vi "GeneratePhaseCUDAv2.vi"() -> ()   [LabVIEW 2019]
uses:
  <vilib>/imath/engines/lvmath2/RunTimeEngine/RangeToken/NIMS_Range.vi
  <instcachedir>/0/NIMS_Range_0856D726B6B24596B614846B21C682A9.lvgen/NIMS_Range_0856D726B6B24596B614846B21C682A9_001.vi
  <vilib>/imath/engines/lvmath2/RunTimeEngine/BuiltInFunctions/meshgrid2d/NIMS_meshgrid2d(V,V).vi
  <instcachedir>/0/NIMS_meshgrid2d(V,V)_3733343E1C554A708015CFB0432C6A59.lvgen/NIMS_meshgrid2d(V,V)_3733343E1C554A708015CFB0432C6A59_000.vi
  <vilib>/imath/engines/lvmath2/RunTimeEngine/ErrorHandling/NIMS_Create Error From Enums.vi
  <vilib>/imath/engines/lvmath2/RunTimeEngine/IndexRead/NIMS M($).vi
  <instcachedir>/0/NIMS M($)_82D1177398184AFB96A6AFB63C3C3F57.lvgen/NIMS M($)_82D1177398184AFB96A6AFB63C3C3F57_000.vi
  <vilib>/imathl/engines/lvmath/Functions/Error Handling/Create Error.vi
  <vilib>/imath/engines/lvmath2/RunTimeEngine/BuiltInFunctions/length/NIMS_length(GV).vi
  <instcachedir>/0/NIMS_length(GV)_08A3D13377FD4E4B96F5795FBF3698FA.lvgen/NIMS_length(GV)_08A3D13377FD4E4B96F5795FBF3698FA_000.vi
  <vilib>/imath/engines/lvmath2/RunTimeEngine/BuiltInFunctions/zeros/NIMS_V=zeros(I32,I32).vi
  <vilib>/imath/engines/lvmath2/RunTimeEngine/BuiltInFunctions/ones/NIMS_V=ones(I32,I32).vi
  <vilib>/imath/engines/lvmath2/RunTimeEngine/NodeEndStatement/NIMS_NodeEndStatement_Output.vi
  <instcachedir>/0/NIMS_NodeEndStatement_Output_53EC0D466D134D7ABD903AC30B43404B.lvgen/NIMS_NodeEndStatement_Output_53EC0D466D134D7ABD903AC30B43404B_005.vi
  <vilib>/imath/engines/lvmath2/RunTimeEngine/ErrorHandling/NIMS_Finalize Error.vi
  PCIe16LabVIEWSDK/Interface.dll
panel:
  out "Delay [ms] 2":dbl
  out "board 2":i32
  out "generatePhase Return 2":i32
  in  "I0":dbl=1.0
  in  "y0":i32
  in  "x0":i32
  in  "dy":i32=24
  in  "dx":i32=24
  in  "ny":i32=12
  in  "nx":i32=12
  in  "Generate":bool
  out "Y Array":sgl[](array[numeric])
  out "X Array":sgl[](array[numeric])
  out "board":i32
  in  "Start SLM":bool
  out "Board ID":i32
  out "# of Boards":i32
  in  "SLM":bool
  out "Delay [ms]":dbl
  out "startCuda Return":i32
  out "Init.":bool
  in  "N Iterations":i32=10
  out "N Pixels":i32
  out "SLM Size":i32
  in  "CUDA":bool
  out "stopCUDA Return":i32
  out "generatePhase Return":i32
  out "Path to CUDA DLL":path
  in  "Stop":bool
  out "Phase SLM":T1(plugin-control)
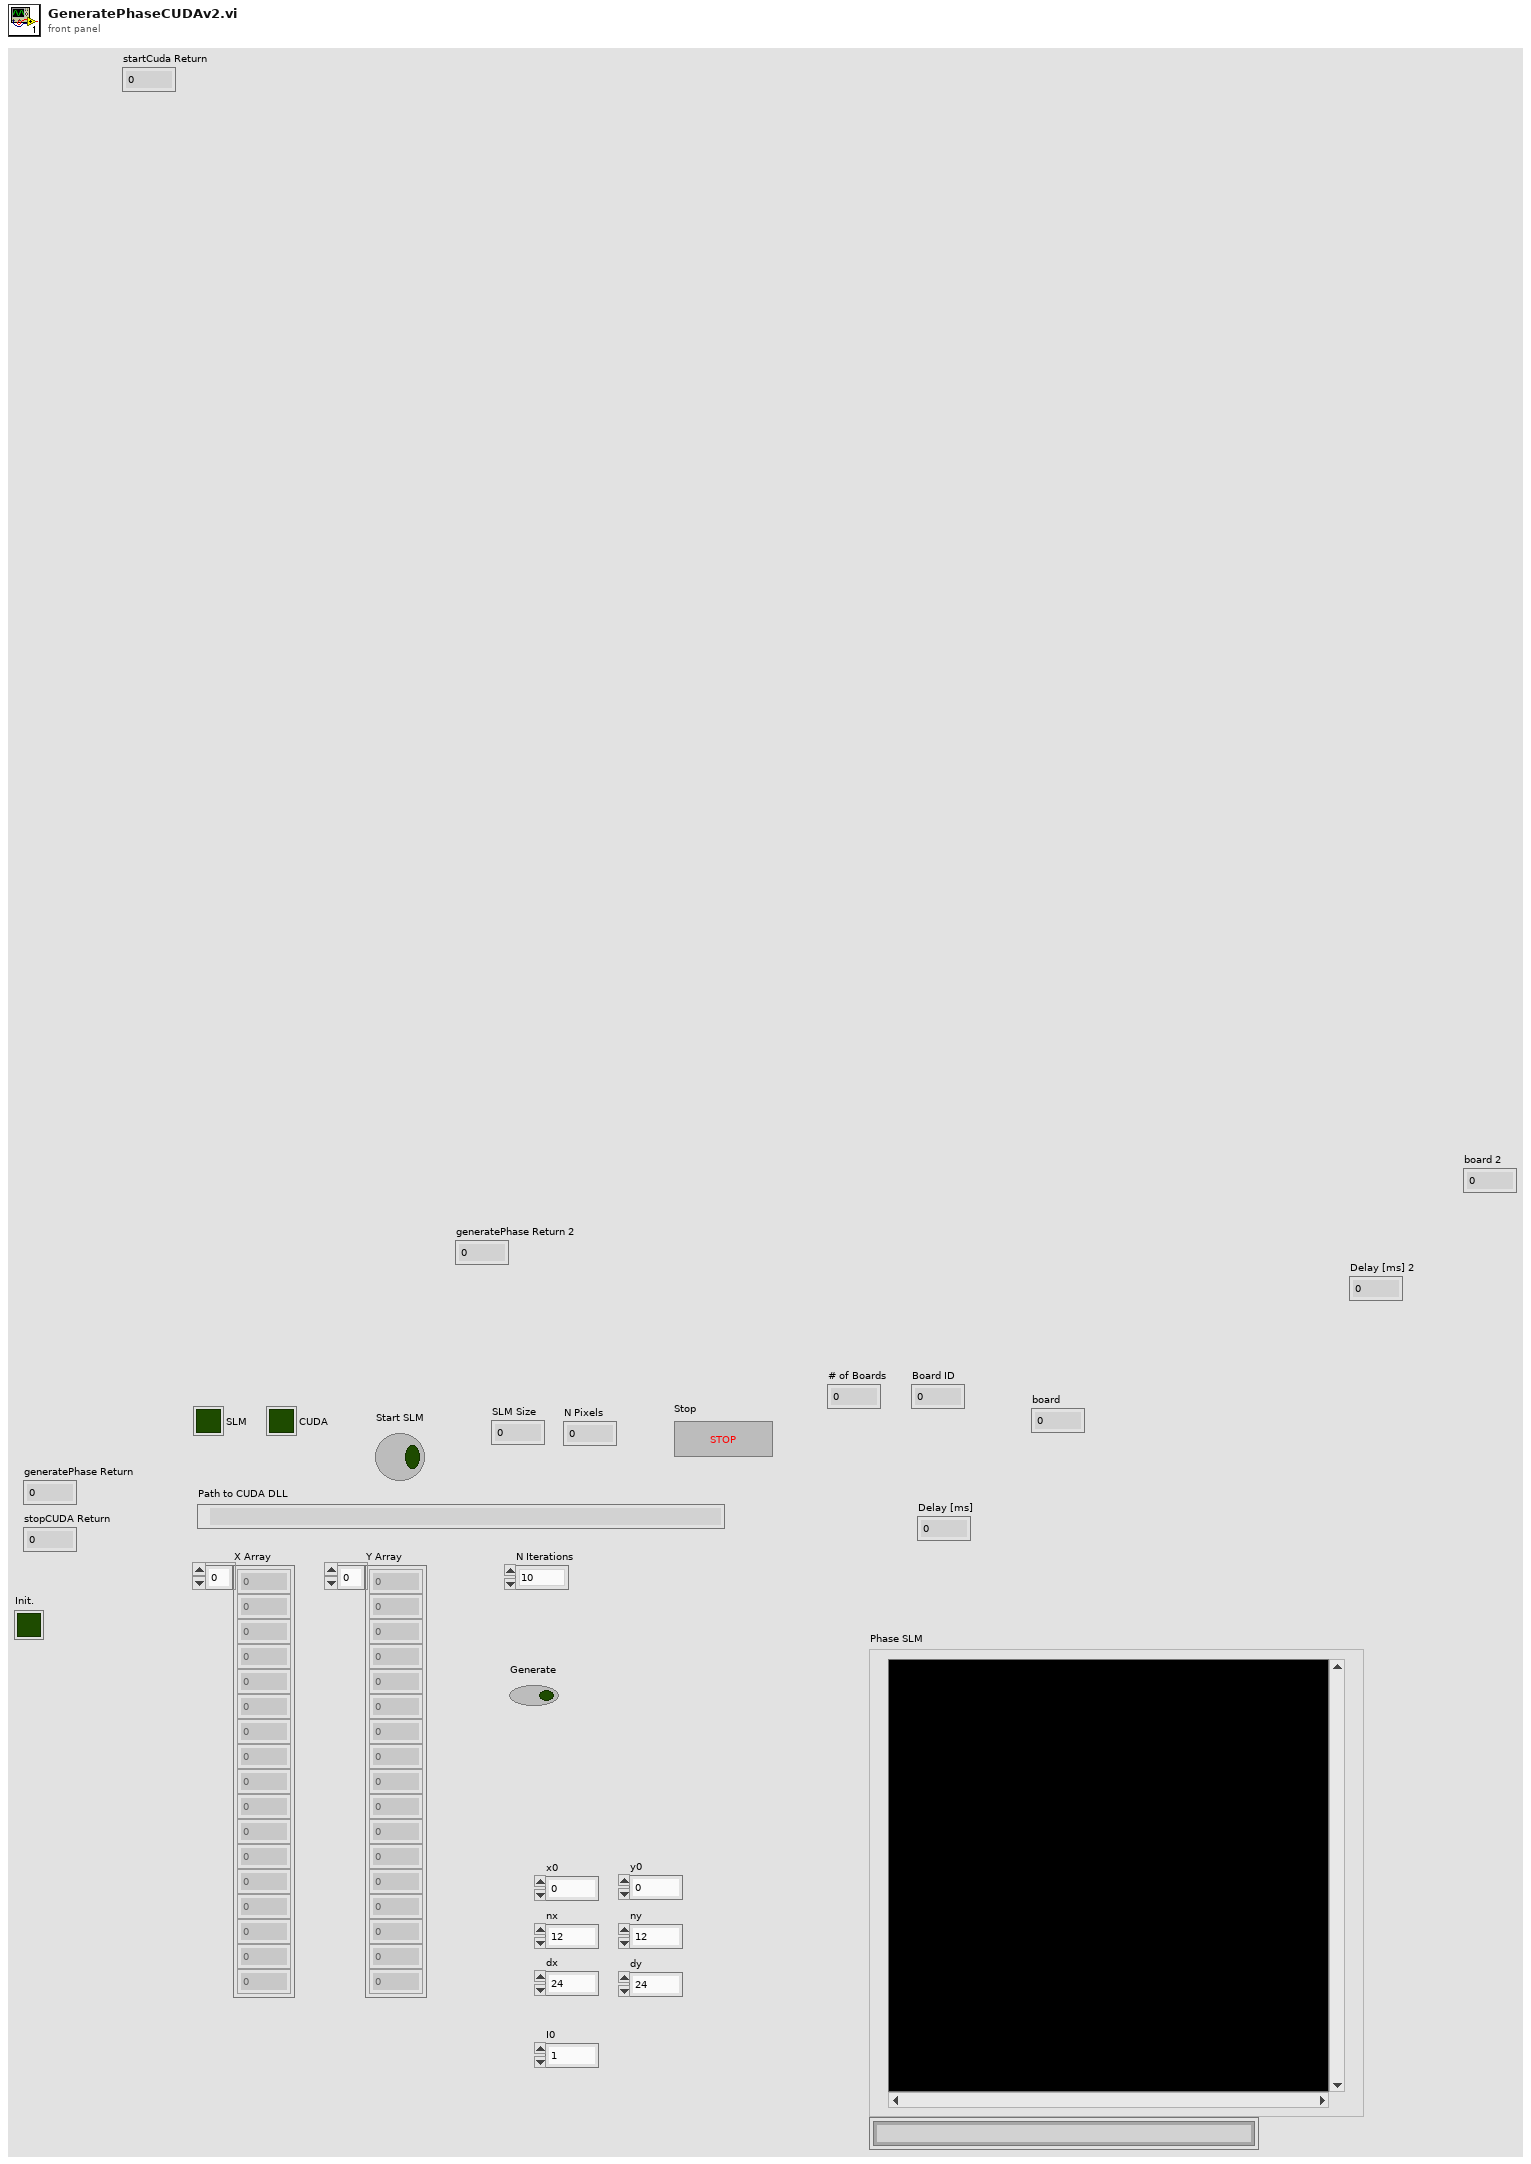
[diagram p1: front panel]
types:
  T1 = typedef "IMAQ Image.ctl" = refnum<image>
  T2 = typedef "Image Type" = u32
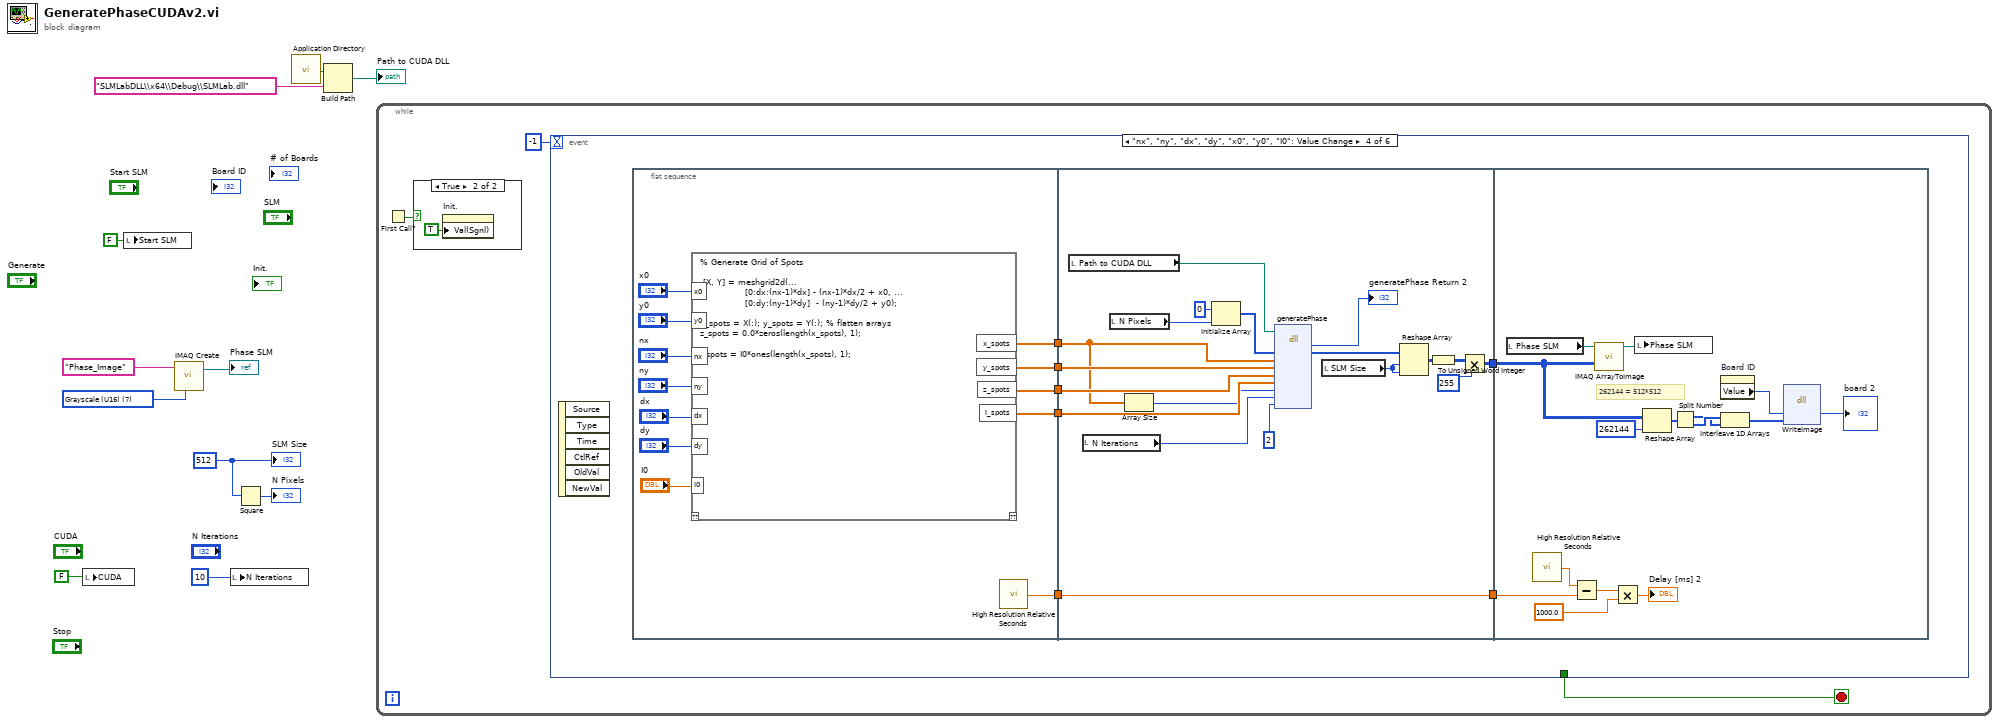
[diagram p0: block diagram]
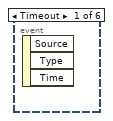
[diagram p3: hidden frame]
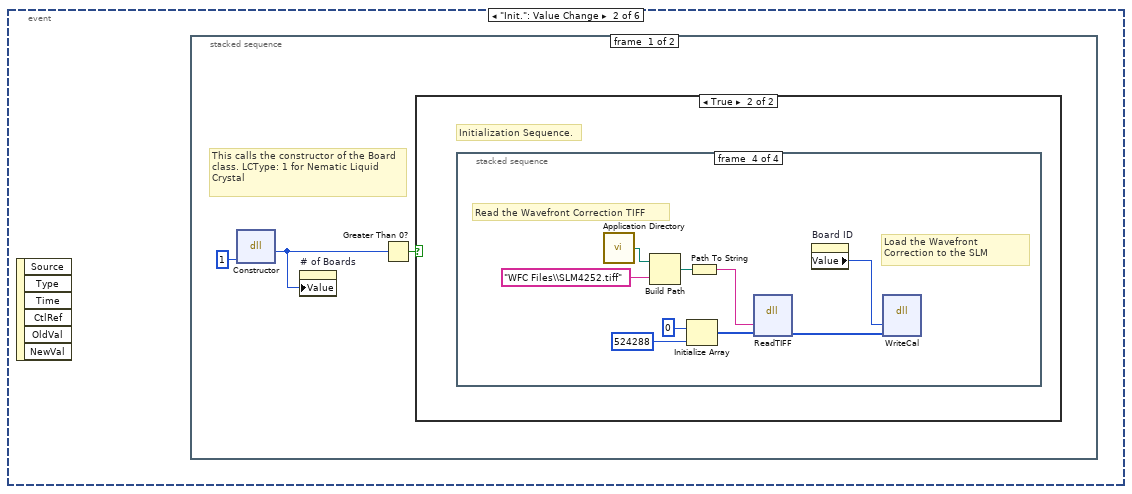
[diagram p4: hidden frame]
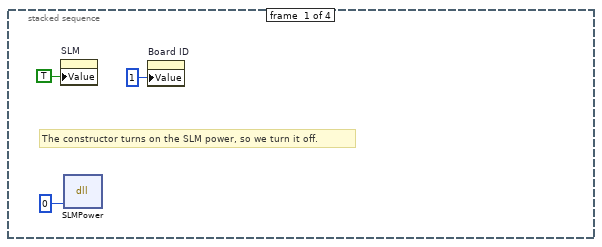
[diagram p6: hidden frame]
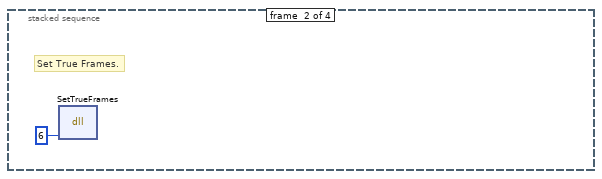
[diagram p7: hidden frame]
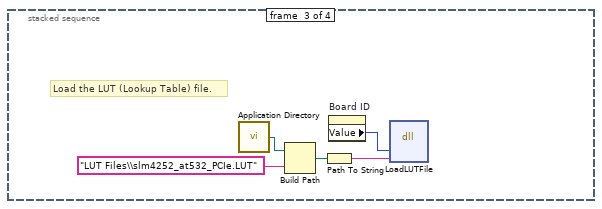
[diagram p8: hidden frame]
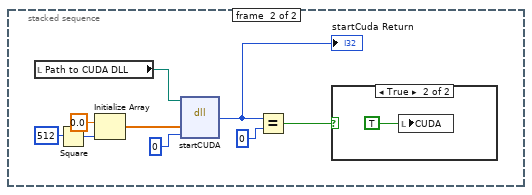
[diagram p9: hidden frame]
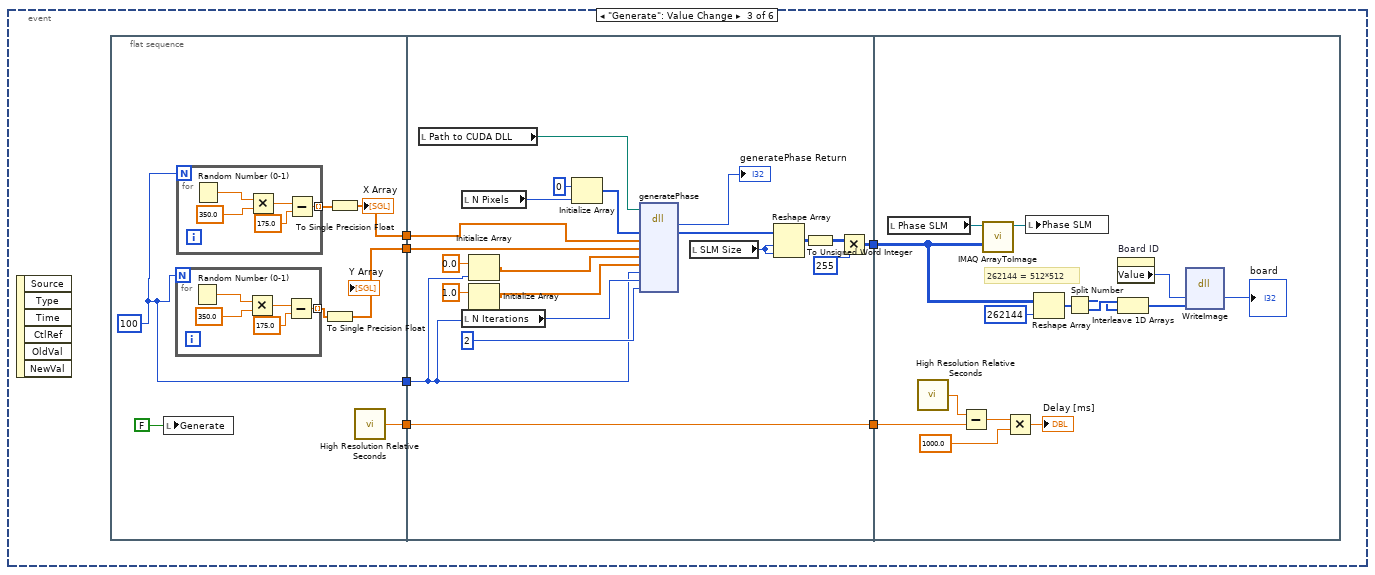
[diagram p11: hidden frame]
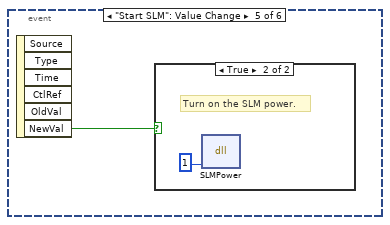
[diagram p12: hidden frame]
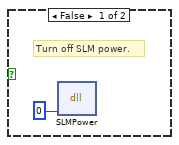
[diagram p13: hidden frame]
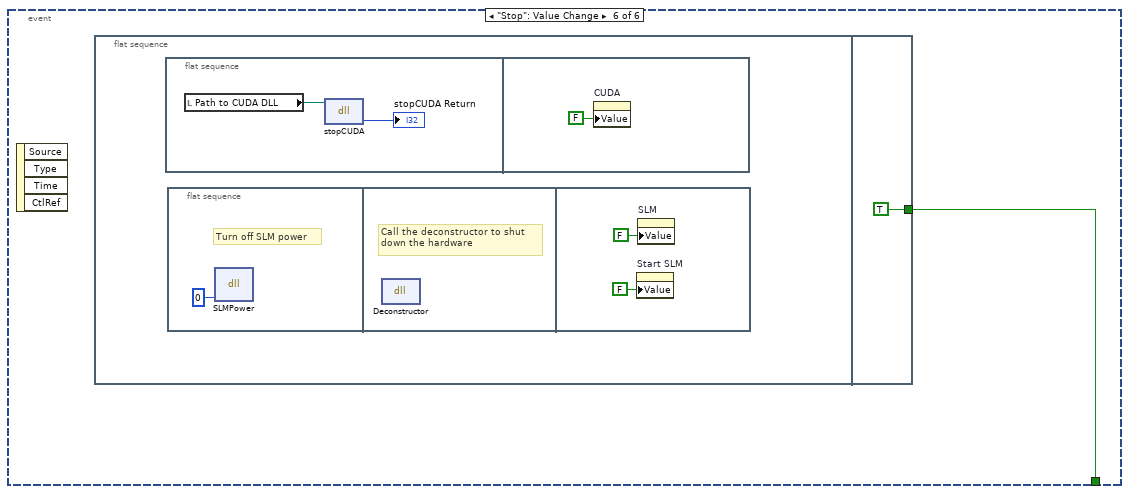
[diagram p14: hidden frame]
diagram:
  w3 = 512
  w10 = T2 7 items=["Grayscale (U8)", "Grayscale (I16)", "Grayscale (SGL)", "Complex (CSG)", "RGB (U32)", "HSL (U32)", "RGB (U64)", "Grayscale (U16)"] ("Image Type")
  n1 = local write "CUDA"(FALSE ("Update SLM")) -> ()
  n2 = local write "Start SLM"(FALSE ("Update SLM")) -> ()
  n3 = call "IMAQ Create"("Image Name"="Phase_Image", "Image Type"=w10) -> ("New Image"=→"Phase SLM":T1)  [unwired: 3 in, 1 out]
  n4 = local write "N Iterations"(10) -> ()
  n5 = Square(x=w3) -> (x^2=→"N Pixels":i32)
  n6 = call <vilib>:"Application Directory.vi"() -> ("Application Directory"=w7:path)
  n7 = Build Path(base path=w7, name or relative path="SLMLabDLL\\x64\\Debug\\SLMLab.dll") -> (appended path=→"Path to CUDA DLL":path)
  n8 = while {
    stop <- w14 stop-if-true
    n9 = First Call?() -> (First Call?: T/F=w12:bool)
    n10 = case shown="True" w12 {
      frame False {
      }
      frame True {
        n11 = property on="Init." class="Bool (strict)"("Val(Sgnl)"=TRUE ("Value (Signaling)")) -> ()  [unwired: 2 in, 2 out]
      }
    }
    n12 = event shown="[3] \"nx\", \"ny\", \"dx\", \"dy\", \"x0\", \"y0\", \"I0\": Value Change" {
      selector: _ -> [_ _ _ _ _ _]
      dyn-events: _ -> [_ _ _ _ _ _]
      timeout: -1 -> [_ _ _ _ _ _]
      tunnel: [_ _ _ _ _ w320] -> w14
      event Timeout {
        n13 = event-data() -> ()  [unwired: 1 in, 3 out]
      }
      event "Init.": Value Change {
        n14 = event-data() -> ()  [unwired: 1 in, 6 out]
        n15 = stacked-sequence {
          frame #0 {
            # "This calls the constructor of the Board class. LCType: 1 for Nematic Liquid Crystal"
            n16 = dll-call lib="C:/PCIe16LabVIEWSDK/Interface.dll" fn="Constructor"("LCType"=u8 1) -> ("return type"=w18:i32)  [unwired: 4 in, 2 out]
            n17 = property on="# of Boards" class="DigNum (strict)"("Value"=w18) -> ()  [unwired: 2 in, 2 out]
            n18 = Greater Than 0?(x=w18) -> (x > 0?=w17:bool)
            n19 = case shown="True" w17 {
              frame False {
              }
              frame True {
                # "Initialization Sequence."
                n20 = stacked-sequence {
                  frame #0 {
                    # "The constructor turns on the SLM power, so we turn it off."
                    n21 = property on="SLM" class="Bool (strict)"("Value"=TRUE ("SLM")) -> ()  [unwired: 2 in, 2 out]
                    n22 = dll-call lib="C:/PCIe16LabVIEWSDK/Interface.dll" fn="SLMPower"("PowerState"=0) -> ()  [unwired: 5 in, 2 out]
                    n23 = property on="Board ID" class="DigNum (strict)"("Value"=1 ("Board Number")) -> ()  [unwired: 2 in, 2 out]
                  }
                  frame #1 {
                    # "Set True Frames."
                    n24 = dll-call lib="C:/PCIe16LabVIEWSDK/Interface.dll" fn="SetTrueFrames"("TrueFrames"=6) -> ()  [unwired: 5 in, 2 out]
                  }
                  frame #2 {
                    # "Load the LUT (Lookup Table) file."
                    n25 = call <vilib>:"Application Directory.vi"() -> ("Application Directory"=w25:path)
                    n26 = Build Path(base path=w25, name or relative path="LUT Files\\slm4252_at532_PCIe.LUT") -> (appended path=w26:path)
                    n27 = Path To String(path=w26) -> (string=w23:string)
                    n28 = property on="Board ID" class="DigNum (strict)"() -> ("Value"=w27:i32)  [unwired: 2 in, 2 out]
                    n29 = dll-call lib="C:/PCIe16LabVIEWSDK/Interface.dll" fn="LoadLUTFile"("board"=w27, "LUTPath"=w23) -> ()  [unwired: 6 in, 2 out]
                  }
                  frame #3 {
                    # "Read the Wavefront Correction TIFF"
                    # "Load the Wavefront Correction to the SLM"
                    n30 = call <vilib>:"Application Directory.vi"() -> ("Application Directory"=w33:path)
                    n31 = Build Path(base path=w33, name or relative path="WFC Files\\SLM4252.tiff") -> (appended path=w34:path)
                    n32 = Initialize Array(u8 0, 524288) -> (w28:u8[])
                    n33 = Path To String(path=w34) -> (string=w31:string)
                    n34 = dll-call lib="C:/PCIe16LabVIEWSDK/Interface.dll" fn="ReadTIFF"("TiffPath"=w31, "Image"=w28) -> ("Image"=w36:u8[])  [unwired: 5 in, 2 out]
                    n35 = property on="Board ID" class="DigNum (strict)"() -> ("Value"=w35:i32)  [unwired: 2 in, 2 out]
                    n36 = dll-call lib="C:/PCIe16LabVIEWSDK/Interface.dll" fn="WriteCal"("board"=w35, "Image"=w36) -> ()  [unwired: 6 in, 2 out]
                  }
                }
              }
            }
          }
          frame #1 {
            n37 = local read "Path to CUDA DLL"() -> (w43:path)
            n38 = Square(x=512 ("dimension size")) -> (x^2=w45:i32)
            n39 = Initialize Array(sgl 0.0 ("element"), w45) -> (w44:sgl[])
            n40 = dll-call lib="?" fn="startCUDA"(path in=w43, "h_pSLMstart"=w44, "deviceID"=0) -> ("Rückgabetyp"=w42:i32)  [unwired: 4 in, 2 out]
            "startCuda Return" <- w42
            n41 = Equal?(x=w42, y=0) -> (x = y?=w41:bool)
            n42 = case shown="True" w41 {
              frame False {
              }
              frame True {
                n43 = local write "CUDA"(TRUE ("Update SLM")) -> ()
              }
            }
          }
        }
      }
      event "Generate": Value Change {
        n44 = event-data() -> ()  [unwired: 1 in, 6 out]
        n45 = flat-sequence {
          tunnel: [w59] -> w51
          tunnel: [w57] -> w49
          tunnel: [w55] -> w48
          tunnel: [w54] -> w47
          tunnel: [w82] -> w52
          tunnel: w51 -> [w82]
          tunnel: [w81] -> w50
          tunnel: w49 -> [w76]
          tunnel: w48 -> [w77]
          tunnel: w47 -> [w70]
          tunnel: w52 -> [w105]
          tunnel: w50 -> [w92]
          frame #0 {
            w54 = 100
            n46 = local write "Generate"(FALSE) -> ()
            n47 = for {
              N: w54 -> [_]
              tunnel: [w60] -> w56 mode=indexing
              n48 = Random Number (0-1)() -> (number: 0 to 1=w64:dbl)
              n49 = Multiply(x=w64, y=350.0) -> (x*y=w62:dbl)
              n50 = Subtract(x=w62, y=175.0) -> (x-y=w60:dbl)
            }
            n51 = for {
              N: w54 -> [_]
              tunnel: [w65] -> w58 mode=indexing
              n52 = Random Number (0-1)() -> (number: 0 to 1=w69:dbl)
              n53 = Multiply(x=w69, y=350.0) -> (x*y=w67:dbl)
              n54 = Subtract(x=w67, y=175.0) -> (x-y=w65:dbl)
            }
            n55 = To Single Precision Float(number=w56) -> (single precision float=w55:sgl[])
            "Y Array" <- w55
            n56 = To Single Precision Float(number=w58) -> (single precision float=w57:sgl[])
            "X Array" <- w57
            n57 = call <vilib>:"High Resolution Relative Seconds.vi"() -> ("relative seconds"=w59:dbl)
          }
          frame #1 {
            n58 = local read "Path to CUDA DLL"() -> (w87:path)
            n59 = local read "N Pixels"() -> (w88:i32)
            n60 = local read "N Iterations"() -> (w90:i32)
            n61 = Initialize Array(sgl 0.0 ("element"), w70) -> (w75:sgl[])
            n62 = Initialize Array(sgl 1.0 ("element"), w70) -> (w71:sgl[])
            n63 = Initialize Array(u8 0 ("element"), w88) -> (w86:u8[])
            n64 = dll-call lib="?" fn="generatePhase"(path in=w87, "h_pSLM_uint16"=w86, "x_spots"=w76, "y_spots"=w77, "z_spots"=w75, "I_spots"=w71, "N_spots"=w70, "N_interations"=w90, "method"=2) -> ("Return Value"=→"generatePhase Return":i32, "h_pSLM_uint16"=w85:u8[])  [unwired: 9 in, 2 out]
            n65 = local read "SLM Size"() -> (w89:i32)
            n66 = Reshape Array(w85, w89, w89) -> (w80:u8[][])
            n67 = To Unsigned Word Integer(number=w80) -> (unsigned 16bit integer=w79:u16[][])
            n68 = Multiply(x=w79, y=u16 255) -> (x*y=w81:u16[][])
          }
          frame #2 {
            # "262144 = 512*512"
            n69 = local read "Phase SLM"() -> (w99:T1)
            n70 = call <vilib>:"High Resolution Relative Seconds.vi"() -> ("relative seconds"=w104:dbl)
            n71 = Subtract(x=w104, y=w105) -> (x-y=w103:dbl)
            n72 = call "IMAQ ArrayToImage"("Image Pixels (U16)"=w92, "Image"=w99) -> ("Image Out"=w100:T1)  [unwired: 8 in, 1 out]
            n73 = Multiply(x=w103, y=1000.0) -> (x*y=→"Delay [ms]":dbl)
            n74 = local write "Phase SLM"(w100) -> ()
            n75 = Reshape Array(w92, 262144 ("dimension size")) -> (w97:u16[])
            n76 = Split Number(x=w97) -> (hi(x)=w94:u8[], lo(x)=w95:u8[])
            n77 = property on="Board ID" class="DigNum (strict)"() -> ("Value"=w98:i32)  [unwired: 2 in, 2 out]
            n78 = Interleave 1D Arrays(w95, w94) -> (w96:u8[])
            n79 = dll-call lib="C:/PCIe16LabVIEWSDK/Interface.dll" fn="WriteImage"("board"=w98, "Image"=w96) -> ("board"=→"board":i32)  [unwired: 5 in, 2 out]
          }
        }
      }
      event "nx", "ny", "dx", "dy", "x0", "y0", "I0": Value Change {
        n80 = event-data() -> ()  [unwired: 1 in, 6 out]
        n81 = flat-sequence {
          tunnel: [w124] -> w112
          tunnel: [w116] -> w111
          tunnel: [w115] -> w110
          tunnel: [w114] -> w109
          tunnel: [w113] -> w108
          tunnel: [w293] -> w107
          tunnel: w112 -> [w293]
          tunnel: [w292] -> w106
          tunnel: w111 -> [w284]
          tunnel: w110 -> [w288]
          tunnel: w109 -> [w286]
          tunnel: w108 -> [w285]
          tunnel: w107 -> [w316]
          tunnel: w106 -> [w303]
          frame #0 {
            n82 = mathscript code="% Generate Grid of Spots\n\n [X, Y] = meshgrid2d(...\n               [0:dx:(nx-1)*dx] - (nx-1)*dx/2 + x0, ...\n               [0:dy:(ny-1)*dy]  - (ny-1)*dy/2 + y0);\n\nx_spots = X(:); y_spots = Y(:); % flatten arrays\nz_spots = 0.0*zeros(length(x_spots), 1);\n\nI_spots = I0*ones(length(x_spots), 1);"("nx"="nx", "ny"="ny", "dx"="dx", "dy"="dy", "x0"="x0", "y0"="y0", "I0"="I0") -> ("x_spots"=w116:dbl[], "y_spots"=w115:dbl[], "I_spots"=w113:dbl[], "z_spots"=w114:dbl[])  [unwired: 1 in, 1 out]
            n83 = call <vilib>:"High Resolution Relative Seconds.vi"() -> ("relative seconds"=w124:dbl)
          }
          frame #1 {
            n84 = local read "Path to CUDA DLL"() -> (w298:path)
            n85 = local read "N Iterations"() -> (w301:i32)
            n86 = local read "N Pixels"() -> (w299:i32)
            n87 = Array Size(array=w284) -> (size(s)=w283:i32)
            n88 = Initialize Array(u8 0 ("element"), w299) -> (w297:u8[])
            n89 = dll-call lib="?" fn="generatePhase"(path in=w298, "h_pSLM_uint16"=w297, "x_spots"=w284, "y_spots"=w288, "z_spots"=w286, "I_spots"=w285, "N_spots"=w283, "N_interations"=w301, "method"=2) -> ("Return Value"=→"generatePhase Return 2":i32, "h_pSLM_uint16"=w296:u8[])  [unwired: 9 in, 2 out]
            n90 = local read "SLM Size"() -> (w300:i32)
            n91 = Reshape Array(w296, w300, w300) -> (w291:u8[][])
            n92 = To Unsigned Word Integer(number=w291) -> (unsigned 16bit integer=w290:u16[][])
            n93 = Multiply(x=w290, y=u16 255) -> (x*y=w292:u16[][])
          }
          frame #2 {
            # "262144 = 512*512"
            n94 = local read "Phase SLM"() -> (w310:T1)
            n95 = call <vilib>:"High Resolution Relative Seconds.vi"() -> ("relative seconds"=w315:dbl)
            n96 = Subtract(x=w315, y=w316) -> (x-y=w314:dbl)
            n97 = call "IMAQ ArrayToImage"("Image Pixels (U16)"=w303, "Image"=w310) -> ("Image Out"=w311:T1)  [unwired: 8 in, 1 out]
            n98 = Multiply(x=w314, y=1000.0) -> (x*y=→"Delay [ms] 2":dbl)
            n99 = local write "Phase SLM"(w311) -> ()
            n100 = Reshape Array(w303, 262144 ("dimension size")) -> (w308:u16[])
            n101 = Split Number(x=w308) -> (hi(x)=w305:u8[], lo(x)=w306:u8[])
            n102 = property on="Board ID" class="DigNum (strict)"() -> ("Value"=w309:i32)  [unwired: 2 in, 2 out]
            n103 = Interleave 1D Arrays(w306, w305) -> (w307:u8[])
            n104 = dll-call lib="C:/PCIe16LabVIEWSDK/Interface.dll" fn="WriteImage"("board"=w309, "Image"=w307) -> ("board"=→"board 2":i32)  [unwired: 5 in, 2 out]
          }
        }
      }
      event "Start SLM": Value Change {
        n105 = event-data() -> ("NewVal"=w317:bool)  [unwired: 1 in, 5 out]
        n106 = case shown="True" w317 {
          frame False {
            # "Turn off SLM power."
            n107 = dll-call lib="C:/PCIe16LabVIEWSDK/Interface.dll" fn="SLMPower"("PowerState"=0) -> ()  [unwired: 5 in, 2 out]
          }
          frame True {
            # "Turn on the SLM power."
            n108 = dll-call lib="C:/PCIe16LabVIEWSDK/Interface.dll" fn="SLMPower"("PowerState"=1) -> ()  [unwired: 5 in, 2 out]
          }
        }
      }
      event "Stop": Value Change {
        n109 = event-data() -> ()  [unwired: 1 in, 4 out]
        n110 = flat-sequence {
          tunnel: [TRUE] -> w320
          frame #0 {
            n111 = flat-sequence {
              frame #0 {
                n112 = local read "Path to CUDA DLL"() -> (w321:path)
                n113 = dll-call lib="?" fn="stopCUDA"(path in=w321) -> ("Return Value"=→"stopCUDA Return":i32)  [unwired: 2 in, 2 out]
              }
              frame #1 {
                n114 = property on="CUDA" class="Bool (strict)"("Value"=FALSE ("SLM")) -> ()  [unwired: 2 in, 2 out]
              }
            }
            n115 = flat-sequence {
              frame #0 {
                # "Turn off SLM power"
                n116 = dll-call lib="C:/PCIe16LabVIEWSDK/Interface.dll" fn="SLMPower"("PowerState"=0) -> ()  [unwired: 5 in, 2 out]
              }
              frame #1 {
                # "Call the deconstructor to shut \ndown the hardware"
                n117 = dll-call lib="C:/PCIe16LabVIEWSDK/Interface.dll" fn="Deconstructor"() -> ()  [unwired: 4 in, 2 out]
              }
              frame #2 {
                n118 = property on="Start SLM" class="Bool (strict)"("Value"=FALSE ("SLM")) -> ()  [unwired: 2 in, 2 out]
                n119 = property on="SLM" class="Bool (strict)"("Value"=FALSE ("SLM")) -> ()  [unwired: 2 in, 2 out]
              }
            }
          }
          frame #1 {
          }
        }
      }
    }
  }
  "SLM Size" <- w3
